vi "switch on request.vi"(8 "Z4(AutoSetState)":T1(array[ring])=[enum."stop ready", enum."stop ready", enum."stop ready", enum."stop ready"], 9 "Z4_tmp(AutoSetState)":T1(array[ring])=[enum."stop ready", enum."stop ready", enum."stop ready", enum."stop ready"], 10 "Z3(State)":T1(array[ring])=[enum."stop ready", enum."stop ready", enum."stop ready", enum."stop ready"], 11 "Z1(CmdSource)":T2(array[ring])=[enum."auto", enum."auto", enum."auto", enum."auto"]) -> (1 "N":i32, 2 "ok":bool, 3 "Z4_out(AutoSetState)":T1(array[ring])=[enum."stop ready", enum."stop ready", enum."stop ready", enum."stop ready"])   [LabVIEW 2019, in "Userlib.lvlib"]
uses:
  Userlib.lvlib
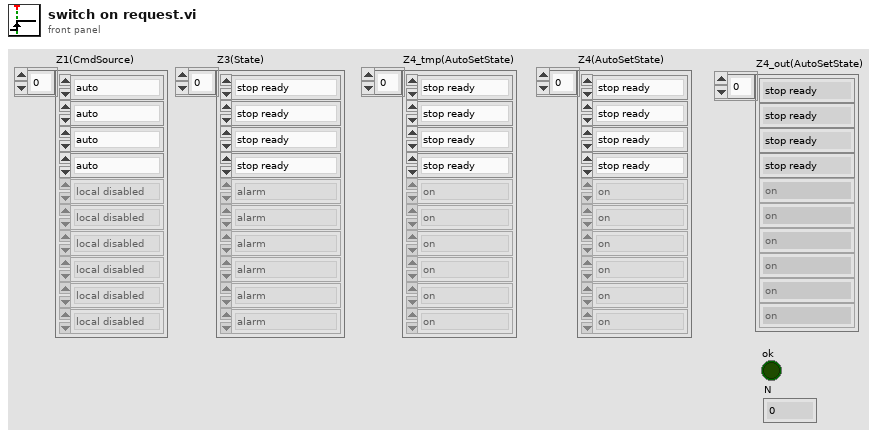
[diagram p1: front panel]
types:
  T1 = enum32{"alarm", "disabled", "not ready", "stop ready", "reserv", "switched off", "switched on", "check", "on min", "decrease speed", "on", "increase speed", "on max"}[]
  T2 = enum32{"local disabled", "local hand", "hand", "auto", "dist"}[]
  T3 = enum32{"alarm", "disabled", "not ready", "stop ready", "reserv", "switched off", "switched on", "check", "on min", "decrease speed", "on", "increase speed", "on max"}
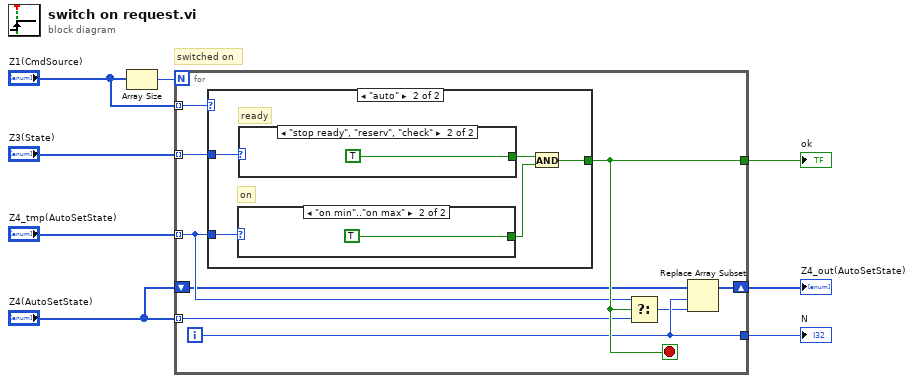
[diagram p0: block diagram]
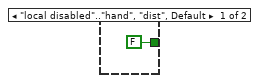
[diagram p2: hidden frame]
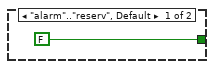
[diagram p3: hidden frame]
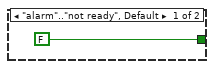
[diagram p4: hidden frame]
diagram:
  # "switched on"
  n1 = Array Size(array="Z1(CmdSource)") -> (size(s)=w6:i32)
  n2 = for {
    N: w6 -> [_]
    tunnel: "Z3(State)" -> [w17] mode=indexing
    tunnel: "Z1(CmdSource)" -> [w16] mode=indexing
    tunnel: [w11] -> w4
    tunnel: "Z4_tmp(AutoSetState)" -> [w14] mode=indexing
    tunnel: [w15] -> w3
    tunnel: "Z4(AutoSetState)" -> [w13] mode=indexing
    shift-right: [w9] -> w2
    shift-left: "Z4(AutoSetState)" -> [w12]
    i -> [w11]
    stop <- w15 stop-if-true
    n3 = case shown="\"auto\"" w16 {
      tunnel: w17 -> [_ w23]
      tunnel: w14 -> [_ w22]
      tunnel: [FALSE w19] -> w15
      frame "local disabled".."hand", "dist", Default {
      }
      frame "auto" {
        # "on"
        # "ready"
        n4 = case shown="\"on min\"..\"on max\"" w22 {
          tunnel: [FALSE TRUE] -> w20
          frame "alarm".."reserv", Default {
          }
          frame "on min".."on max" {
          }
        }
        n5 = case shown="\"stop ready\", \"reserv\", \"check\"" w23 {
          tunnel: [FALSE TRUE] -> w21
          frame "alarm".."not ready", Default {
          }
          frame "stop ready", "reserv", "check" {
          }
        }
        n6 = And(x=w21, y=w20) -> (x .and. y?=w19:bool)
      }
    }
    n7 = Select(t=w14, s=w15, f=w13) -> (s? t:f=w10:T3)
    n8 = Replace Array Subset(array=w12, new element=w10, index=w11) -> (w9:T1)
  }
  "Z4_out(AutoSetState)" <- w2
  "N" <- w4
  "ok" <- w3
